vi "Read Data.vi"(11 "Data Update Msg in":refnum<class "Data Update Msg.lvclass">) -> (2 "Data":cluster{"EDR":dbl, "Pulse":u8}, 3 "Data Update Msg out":refnum<class "Data Update Msg.lvclass">)   [LabVIEW 2011, in "Data Update Msg.lvclass"]
uses:
  Data Update Msg.lvclass
  Data Update Msg.lvclass/Data Update Msg.ctl
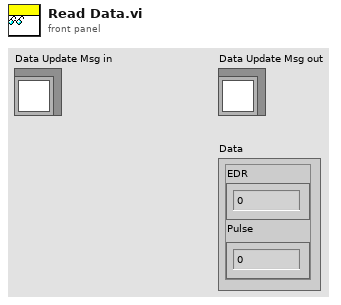
[diagram p1: front panel]
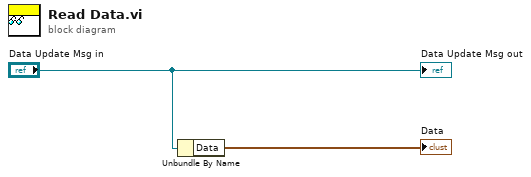
[diagram p0: block diagram]
diagram:
  n1 = Unbundle By Name("Data Update Msg in") -> ("Data"=→"Data":cluster{"EDR":dbl, "Pulse":u8})
  "Data Update Msg out" <- "Data Update Msg in"
